vi "Add Units Panel 2.vi"(0 "System#":u8, 7 "Rack Number":i8=1 min=1 max=16, 8 "AutoAge.ini  File Path":path=path "\\\\Beco\\autoage/config/autoage.ini") -> ()   [LabVIEW 2021]
uses:
  Main Controls System v8.0/AutoAge Globals.vi
panel:
  out "Functional  Data":string
  out "title":string
  in  "Cancel":bool
  in  "Test":bool
  in  "Update":bool
  in  "Row33 to 40":bool
  in  "Row25 to 32":bool
  in  "Row17 to 24":bool
  in  "Row9 to 16":bool
  in  "Row1 to 8":bool
  in  "Select All":bool
  in  "40":bool
  in  "39":bool
  in  "38":bool
  in  "37":bool
  in  "36":bool
  in  "35":bool
  in  "34":bool
  in  "33":bool
  in  "32":bool
  in  "31":bool
  in  "30":bool
  in  "29":bool
  in  "28":bool
  in  "27":bool
  in  "26":bool
  in  "25":bool
  in  "24":bool
  in  "23":bool
  in  "22":bool
  in  "21":bool
  in  "20":bool
  in  "19":bool
  in  "18":bool
  in  "17":bool
  in  "16":bool
  in  "15":bool
  in  "14":bool
  in  "13":bool
  in  "12":bool
  in  "11":bool
  in  "10":bool
  in  "9":bool
  in  "8":bool
  in  "7":bool
  in  "6":bool
  in  "5":bool
  in  "4":bool
  in  "3":bool
  in  "2":bool
  in  "1":bool
  out "Rack":i8=1 min=1 max=16
  in  "Done":bool
  # "Click to turn on the inactive positions.  A red square   in a position indicates that a position is going to run."
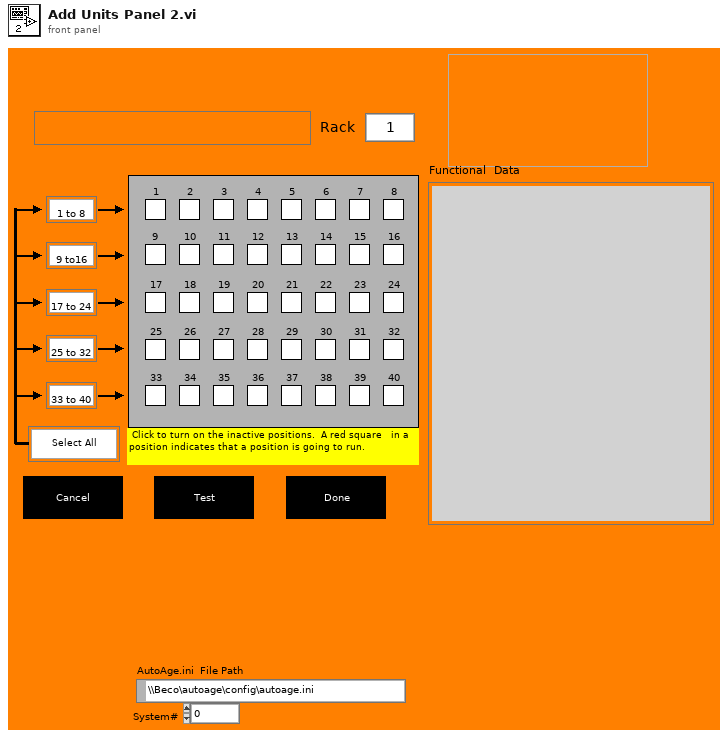
[diagram p1: front panel]
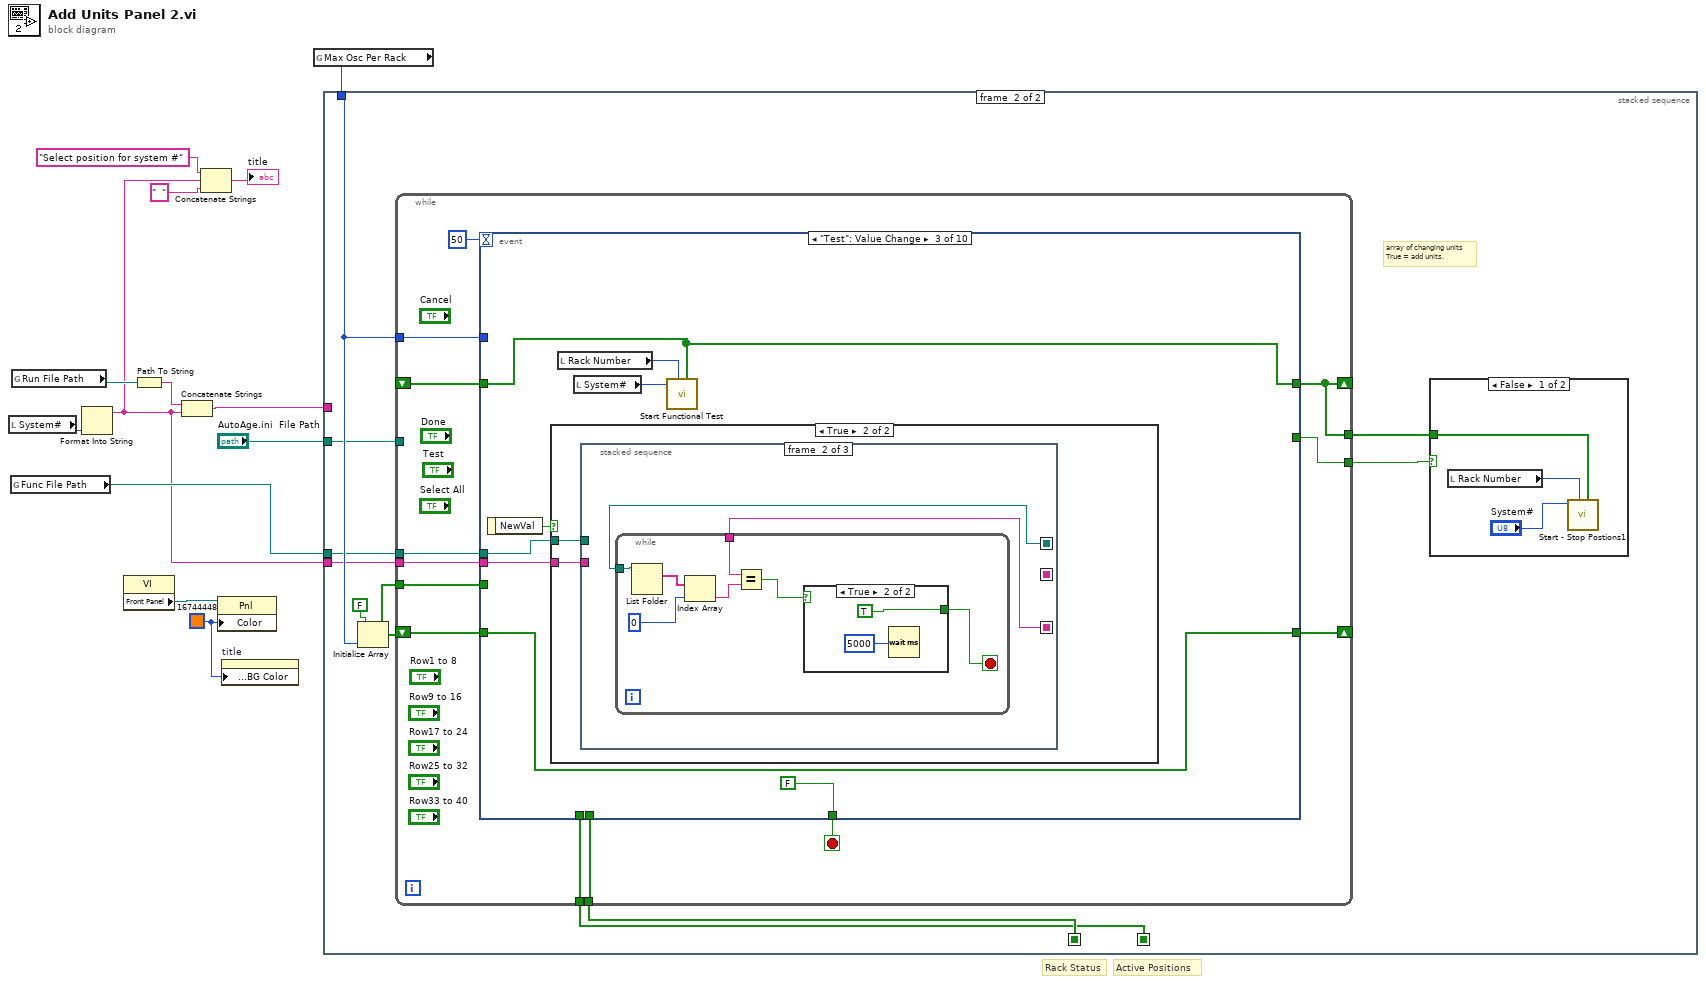
[diagram p0: block diagram]
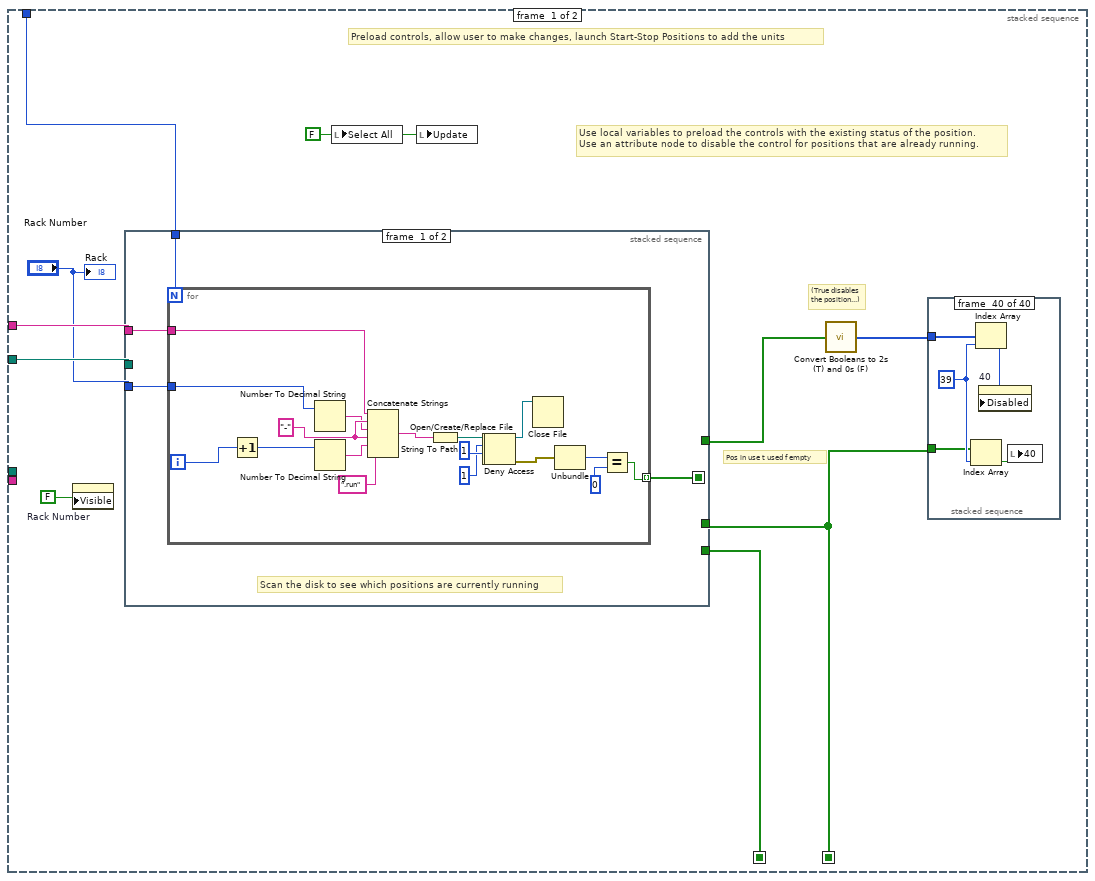
[diagram p2: hidden frame]
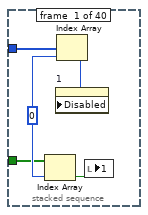
[diagram p3: hidden frame]
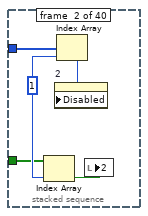
[diagram p4: hidden frame]
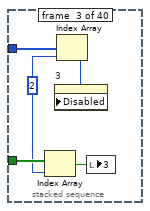
[diagram p5: hidden frame]
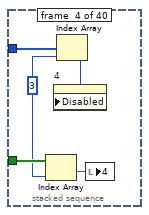
[diagram p6: hidden frame]
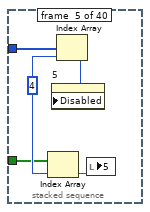
[diagram p7: hidden frame]
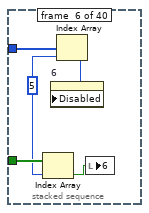
[diagram p8: hidden frame]
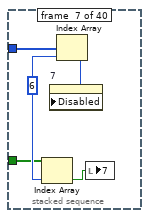
[diagram p9: hidden frame]
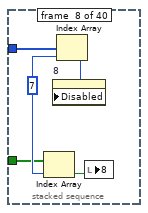
[diagram p10: hidden frame]
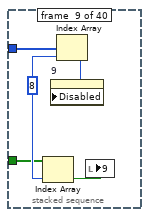
[diagram p11: hidden frame]
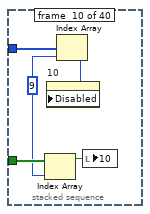
[diagram p12: hidden frame]
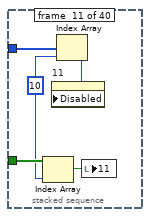
[diagram p13: hidden frame]
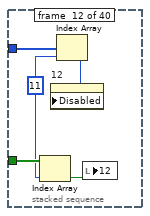
[diagram p14: hidden frame]
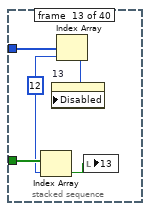
[diagram p15: hidden frame]
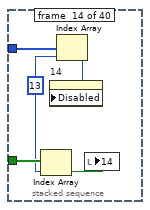
[diagram p16: hidden frame]
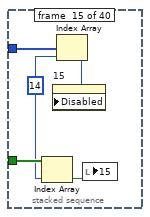
[diagram p17: hidden frame]
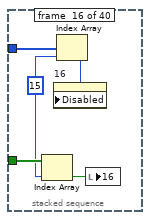
[diagram p18: hidden frame]
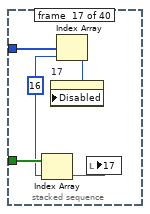
[diagram p19: hidden frame]
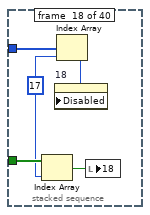
[diagram p20: hidden frame]
diagram:
  w1 = u32 16744448
  # "Active Positions"
  # "Rack Status"
  n1 = local read "System#"() -> (w11:u8)
  n2 = global read "AutoAge Globals.vi" "Func File Path"() -> (w7:path)
  n3 = global read "AutoAge Globals.vi" "Run File Path"() -> (w12:path)
  n4 = Format Into String(w11) -> (resulting string=w4:string)  [unwired: 3 in, 1 out]
  n5 = property class="VI"() -> ("Front Panel"=w6:refnum<vi>)  [unwired: 2 in, 2 out]
  n6 = Path To String(path=w12) -> (string=w8:string)
  n7 = Concatenate Strings(w8, w4) -> (w10:string)
  n8 = Concatenate Strings("Select position for system #", w4, "  ") -> (→"title":string)
  n9 = property class="Pnl"(reference=w6, "Color"=w1) -> ()  [unwired: 1 in, 2 out]
  n10 = property on="title" class="Str"("Text.Text Colors:BG Color"=w1) -> ()  [unwired: 2 in, 2 out]
  n11 = global read "AutoAge Globals.vi" "Max Osc Per Rack"() -> (w9:u16)
  n12 = stacked-sequence {
    seq-local: [w19 _] -> [_ w278]
    seq-local: [w14 _] -> [_ w279]
    tunnel: "AutoAge.ini  File Path" -> [w22 w273]
    tunnel: w10 -> [w21 _]
    tunnel: w9 -> [w17 w282]
    tunnel: w7 -> [_ w277]
    tunnel: w4 -> [_ w276]
    frame #0 {
      w16 = FALSE ("Select All")
      # "Pos in use t used f empty"
      # "(True disables\nthe position...)"
      # "Preload controls, allow user to make changes, launch Start-Stop Positions to add the units"
      # "Use local variables to preload the controls with the existing status of the position.\nUse an attribute node to disable the control for positions that are already running."
      n13 = property on="Rack Number" class="DigNum (strict)"("Visible"=FALSE) -> ()  [unwired: 2 in, 2 out]
      n14 = stacked-sequence {
        seq-local: [w227 _] -> [_ w253]
        tunnel: "Rack Number" -> [w226 w261]
        tunnel: [_ w252] -> w15
        tunnel: [_ w253] -> w19
        tunnel: w22 -> [_ w250]
        tunnel: w21 -> [w225 _]
        tunnel: w17 -> [w224 w249]
        tunnel: [_ w247] -> w14
        frame #0 {
          # "Scan the disk to see which positions are currently running"
          n15 = for {
            N: w224 -> [_]
            tunnel: [w231] -> w227 mode=indexing
            tunnel: w226 -> [w233]
            tunnel: w225 -> [w232]
            i -> [w230]
            w246 = "-"
            n16 = Increment(x=w230) -> (x+1=w244:i32)
            n17 = Number To Decimal String(number=w233) -> (decimal integer string=w241:string)  [unwired: 1 in]
            n18 = Number To Decimal String(number=w244) -> (decimal integer string=w242:string)  [unwired: 1 in]
            n19 = Concatenate Strings(w232, w246, w241, w246, w242, ".run") -> (w243:string)
            n20 = String To Path(string=w243) -> (path=w234:path)
            n21 = Open/Create/Replace File(file path (use dialog)=w234, access (0:read/write)=1) -> (refnum out=w228:refnum<file>, error out=w229:errorcluster)  [unwired: 4 in, 1 out]
            n22 = Deny Access(4:w229, 6:1, 7:w228) -> (0:w237:errorcluster, 3:w240:refnum<file>)
            n23 = Close File(refnum=w240) -> ()  [unwired: 1 in, 2 out]
            n24 = Unbundle(w237) -> ("code"=w239:i32)  [unwired: 2 out]
            n25 = Equal?(x=w239, y=0) -> (x = y?=w231:bool)
          }
        }
        frame #1 {
          # "default all pos false"
          # "Resolve card disabled"
          # "resolve rack enabled\nall pos false if disabled"
          # "Check configuration file to see which racks are disabled and how many cards are in each switcher"
          n26 = Decrement(x=w261) -> (x-1=w251:i8)
          n27 = call "Load Rack Config"("AutoAge.ini  File Path"=w250) -> ("Rack Status"=w262:string[], "# of Cards"=w266:i32[])  [unwired: 1 out]
          n28 = Index Array(array=w262, index=w251) -> (element=w260:string)
          n29 = Index Array(array=w266, index=w251) -> (element=w267:i32)
          n30 = Initialize Array(FALSE, w249) -> (w256:bool[])
          n31 = To Lower Case(string=w260) -> (all lower case string=w265:string)
          n32 = Multiply(x=w267, y=8) -> (x*y=w257:i32)
          n33 = for {
            N: w249 -> [_]
            tunnel: w257 -> [w272]
            shift-right: [w269] -> w254
            shift-left: w256 -> [w270]
            i -> [w268]
            n34 = Greater?(x=w272, y=w268) -> (0:w271:bool)
            n35 = Replace Array Subset(array=w270, new element=w271, index=w268) -> (w269:bool[])
          }
          n36 = Equal?(x=w265, y="enabled") -> (x = y?=w259:bool)
          n37 = Initialize Array(w259, w249) -> (w255:bool[])
          n38 = And(x=w255, y=w254) -> (x .and. y?=w247:bool[])
          n39 = Not(x=w247) -> (.not. x?=w248:bool[])
          n40 = Or(x=w248, y=w253) -> (x .or. y?=w252:bool[])
        }
      }
      n41 = local write "Select All"(w16) -> ()
      n42 = local write "Update"(w16) -> ()
      n43 = call "Convert Booleans to 2s (T) and 0s (F)"("Boolean Array"=w15) -> ("2s and 0s"=w18:u8[])
      n44 = stacked-sequence {
        tunnel: w18 -> [w28 w33 w38 w43 w48 w53 w58 w63 w68 w73 w78 w83 w88 w93 w98 w103 w108 w113 w118 w123 w128 w133 w138 w143 w148 w153 w158 w163 w168 w173 w178 w183 w188 w193 w198 w203 w208 w213 w218 w223]
        tunnel: w19 -> [w25 w30 w37 w42 w46 w52 w56 w61 w66 w72 w77 w82 w87 w92 w97 w102 w107 w112 w117 w122 w127 w132 w137 w142 w147 w152 w157 w162 w167 w172 w177 w182 w187 w192 w197 w202 w207 w212 w217 w220]
        frame #0 {
          w26 = 0
          n45 = Index Array(array=w25, index=w26) -> (element=w27:bool)
          n46 = Index Array(array=w28, index=w26) -> (element=w24:u8)
          n47 = property on="1" class="Bool (strict)"("Disabled"=w24) -> ()  [unwired: 2 in, 2 out]
          n48 = local write "1"(w27) -> ()
        }
        frame #1 {
          w32 = 1
          n49 = Index Array(array=w30, index=w32) -> (element=w31:bool)
          n50 = Index Array(array=w33, index=w32) -> (element=w29:u8)
          n51 = property on="2" class="Bool (strict)"("Disabled"=w29) -> ()  [unwired: 2 in, 2 out]
          n52 = local write "2"(w31) -> ()
        }
        frame #2 {
          w36 = 2
          n53 = Index Array(array=w37, index=w36) -> (element=w35:bool)
          n54 = Index Array(array=w38, index=w36) -> (element=w34:u8)
          n55 = property on="3" class="Bool (strict)"("Disabled"=w34) -> ()  [unwired: 2 in, 2 out]
          n56 = local write "3"(w35) -> ()
        }
        frame #3 {
          w41 = 3
          n57 = Index Array(array=w42, index=w41) -> (element=w40:bool)
          n58 = Index Array(array=w43, index=w41) -> (element=w39:u8)
          n59 = property on="4" class="Bool (strict)"("Disabled"=w39) -> ()  [unwired: 2 in, 2 out]
          n60 = local write "4"(w40) -> ()
        }
        frame #4 {
          w47 = 4
          n61 = Index Array(array=w46, index=w47) -> (element=w45:bool)
          n62 = Index Array(array=w48, index=w47) -> (element=w44:u8)
          n63 = property on="5" class="Bool (strict)"("Disabled"=w44) -> ()  [unwired: 2 in, 2 out]
          n64 = local write "5"(w45) -> ()
        }
        frame #5 {
          w51 = 5
          n65 = Index Array(array=w52, index=w51) -> (element=w50:bool)
          n66 = Index Array(array=w53, index=w51) -> (element=w49:u8)
          n67 = property on="6" class="Bool (strict)"("Disabled"=w49) -> ()  [unwired: 2 in, 2 out]
          n68 = local write "6"(w50) -> ()
        }
        frame #6 {
          w57 = 6
          n69 = Index Array(array=w56, index=w57) -> (element=w55:bool)
          n70 = Index Array(array=w58, index=w57) -> (element=w54:u8)
          n71 = property on="7" class="Bool (strict)"("Disabled"=w54) -> ()  [unwired: 2 in, 2 out]
          n72 = local write "7"(w55) -> ()
        }
        frame #7 {
          w62 = 7
          n73 = Index Array(array=w61, index=w62) -> (element=w60:bool)
          n74 = Index Array(array=w63, index=w62) -> (element=w59:u8)
          n75 = property on="8" class="Bool (strict)"("Disabled"=w59) -> ()  [unwired: 2 in, 2 out]
          n76 = local write "8"(w60) -> ()
        }
        frame #8 {
          w67 = 8
          n77 = Index Array(array=w66, index=w67) -> (element=w65:bool)
          n78 = Index Array(array=w68, index=w67) -> (element=w64:u8)
          n79 = property on="9" class="Bool (strict)"("Disabled"=w64) -> ()  [unwired: 2 in, 2 out]
          n80 = local write "9"(w65) -> ()
        }
        frame #9 {
          w70 = 9
          n81 = Index Array(array=w72, index=w70) -> (element=w71:bool)
          n82 = Index Array(array=w73, index=w70) -> (element=w69:u8)
          n83 = property on="10" class="Bool (strict)"("Disabled"=w69) -> ()  [unwired: 2 in, 2 out]
          n84 = local write "10"(w71) -> ()
        }
        frame #10 {
          w75 = 10
          n85 = Index Array(array=w77, index=w75) -> (element=w76:bool)
          n86 = Index Array(array=w78, index=w75) -> (element=w74:u8)
          n87 = property on="11" class="Bool (strict)"("Disabled"=w74) -> ()  [unwired: 2 in, 2 out]
          n88 = local write "11"(w76) -> ()
        }
        frame #11 {
          w80 = 11
          n89 = Index Array(array=w82, index=w80) -> (element=w81:bool)
          n90 = Index Array(array=w83, index=w80) -> (element=w79:u8)
          n91 = property on="12" class="Bool (strict)"("Disabled"=w79) -> ()  [unwired: 2 in, 2 out]
          n92 = local write "12"(w81) -> ()
        }
        frame #12 {
          w85 = 12
          n93 = Index Array(array=w87, index=w85) -> (element=w86:bool)
          n94 = Index Array(array=w88, index=w85) -> (element=w84:u8)
          n95 = property on="13" class="Bool (strict)"("Disabled"=w84) -> ()  [unwired: 2 in, 2 out]
          n96 = local write "13"(w86) -> ()
        }
        frame #13 {
          w91 = 13
          n97 = Index Array(array=w92, index=w91) -> (element=w90:bool)
          n98 = Index Array(array=w93, index=w91) -> (element=w89:u8)
          n99 = property on="14" class="Bool (strict)"("Disabled"=w89) -> ()  [unwired: 2 in, 2 out]
          n100 = local write "14"(w90) -> ()
        }
        frame #14 {
          w96 = 14
          n101 = Index Array(array=w97, index=w96) -> (element=w95:bool)
          n102 = Index Array(array=w98, index=w96) -> (element=w94:u8)
          n103 = property on="15" class="Bool (strict)"("Disabled"=w94) -> ()  [unwired: 2 in, 2 out]
          n104 = local write "15"(w95) -> ()
        }
        frame #15 {
          w101 = 15
          n105 = Index Array(array=w102, index=w101) -> (element=w100:bool)
          n106 = Index Array(array=w103, index=w101) -> (element=w99:u8)
          n107 = property on="16" class="Bool (strict)"("Disabled"=w99) -> ()  [unwired: 2 in, 2 out]
          n108 = local write "16"(w100) -> ()
        }
        frame #16 {
          w106 = 16
          n109 = Index Array(array=w107, index=w106) -> (element=w105:bool)
          n110 = Index Array(array=w108, index=w106) -> (element=w104:u8)
          n111 = property on="17" class="Bool (strict)"("Disabled"=w104) -> ()  [unwired: 2 in, 2 out]
          n112 = local write "17"(w105) -> ()
        }
        frame #17 {
          w111 = 17
          n113 = Index Array(array=w112, index=w111) -> (element=w110:bool)
          n114 = Index Array(array=w113, index=w111) -> (element=w109:u8)
          n115 = property on="18" class="Bool (strict)"("Disabled"=w109) -> ()  [unwired: 2 in, 2 out]
          n116 = local write "18"(w110) -> ()
        }
        frame #18 {
          w116 = 18
          n117 = Index Array(array=w117, index=w116) -> (element=w115:bool)
          n118 = Index Array(array=w118, index=w116) -> (element=w114:u8)
          n119 = property on="19" class="Bool (strict)"("Disabled"=w114) -> ()  [unwired: 2 in, 2 out]
          n120 = local write "19"(w115) -> ()
        }
        frame #19 {
          w121 = 19
          n121 = Index Array(array=w122, index=w121) -> (element=w120:bool)
          n122 = Index Array(array=w123, index=w121) -> (element=w119:u8)
          n123 = property on="20" class="Bool (strict)"("Disabled"=w119) -> ()  [unwired: 2 in, 2 out]
          n124 = local write "20"(w120) -> ()
        }
        frame #20 {
          w125 = 20
          n125 = Index Array(array=w127, index=w125) -> (element=w126:bool)
          n126 = Index Array(array=w128, index=w125) -> (element=w124:u8)
          n127 = property on="21" class="Bool (strict)"("Disabled"=w124) -> ()  [unwired: 2 in, 2 out]
          n128 = local write "21"(w126) -> ()
        }
        frame #21 {
          w131 = 21
          n129 = Index Array(array=w132, index=w131) -> (element=w130:bool)
          n130 = Index Array(array=w133, index=w131) -> (element=w129:u8)
          n131 = property on="22" class="Bool (strict)"("Disabled"=w129) -> ()  [unwired: 2 in, 2 out]
          n132 = local write "22"(w130) -> ()
        }
        frame #22 {
          w136 = 22
          n133 = Index Array(array=w137, index=w136) -> (element=w135:bool)
          n134 = Index Array(array=w138, index=w136) -> (element=w134:u8)
          n135 = property on="23" class="Bool (strict)"("Disabled"=w134) -> ()  [unwired: 2 in, 2 out]
          n136 = local write "23"(w135) -> ()
        }
        frame #23 {
          w141 = 23
          n137 = Index Array(array=w142, index=w141) -> (element=w140:bool)
          n138 = Index Array(array=w143, index=w141) -> (element=w139:u8)
          n139 = property on="24" class="Bool (strict)"("Disabled"=w139) -> ()  [unwired: 2 in, 2 out]
          n140 = local write "24"(w140) -> ()
        }
        frame #24 {
          w146 = 24
          n141 = Index Array(array=w147, index=w146) -> (element=w145:bool)
          n142 = Index Array(array=w148, index=w146) -> (element=w144:u8)
          n143 = property on="25" class="Bool (strict)"("Disabled"=w144) -> ()  [unwired: 2 in, 2 out]
          n144 = local write "25"(w145) -> ()
        }
        frame #25 {
          w151 = 25
          n145 = Index Array(array=w152, index=w151) -> (element=w150:bool)
          n146 = Index Array(array=w153, index=w151) -> (element=w149:u8)
          n147 = property on="26" class="Bool (strict)"("Disabled"=w149) -> ()  [unwired: 2 in, 2 out]
          n148 = local write "26"(w150) -> ()
        }
        frame #26 {
          w156 = 26
          n149 = Index Array(array=w157, index=w156) -> (element=w155:bool)
          n150 = Index Array(array=w158, index=w156) -> (element=w154:u8)
          n151 = property on="27" class="Bool (strict)"("Disabled"=w154) -> ()  [unwired: 2 in, 2 out]
          n152 = local write "27"(w155) -> ()
        }
        frame #27 {
          w161 = 27
          n153 = Index Array(array=w162, index=w161) -> (element=w160:bool)
          n154 = Index Array(array=w163, index=w161) -> (element=w159:u8)
          n155 = property on="28" class="Bool (strict)"("Disabled"=w159) -> ()  [unwired: 2 in, 2 out]
          n156 = local write "28"(w160) -> ()
        }
        frame #28 {
          w166 = 28
          n157 = Index Array(array=w167, index=w166) -> (element=w165:bool)
          n158 = Index Array(array=w168, index=w166) -> (element=w164:u8)
          n159 = property on="29" class="Bool (strict)"("Disabled"=w164) -> ()  [unwired: 2 in, 2 out]
          n160 = local write "29"(w165) -> ()
        }
        frame #29 {
          w171 = 29
          n161 = Index Array(array=w172, index=w171) -> (element=w170:bool)
          n162 = Index Array(array=w173, index=w171) -> (element=w169:u8)
          n163 = property on="30" class="Bool (strict)"("Disabled"=w169) -> ()  [unwired: 2 in, 2 out]
          n164 = local write "30"(w170) -> ()
        }
        frame #30 {
          w176 = 30
          n165 = Index Array(array=w177, index=w176) -> (element=w175:bool)
          n166 = Index Array(array=w178, index=w176) -> (element=w174:u8)
          n167 = property on="31" class="Bool (strict)"("Disabled"=w174) -> ()  [unwired: 2 in, 2 out]
          n168 = local write "31"(w175) -> ()
        }
        frame #31 {
          w181 = 31
          n169 = Index Array(array=w182, index=w181) -> (element=w180:bool)
          n170 = Index Array(array=w183, index=w181) -> (element=w179:u8)
          n171 = property on="32" class="Bool (strict)"("Disabled"=w179) -> ()  [unwired: 2 in, 2 out]
          n172 = local write "32"(w180) -> ()
        }
        frame #32 {
          w186 = 32
          n173 = Index Array(array=w187, index=w186) -> (element=w185:bool)
          n174 = Index Array(array=w188, index=w186) -> (element=w184:u8)
          n175 = property on="33" class="Bool (strict)"("Disabled"=w184) -> ()  [unwired: 2 in, 2 out]
          n176 = local write "33"(w185) -> ()
        }
        frame #33 {
          w191 = 33
          n177 = Index Array(array=w192, index=w191) -> (element=w190:bool)
          n178 = Index Array(array=w193, index=w191) -> (element=w189:u8)
          n179 = property on="34" class="Bool (strict)"("Disabled"=w189) -> ()  [unwired: 2 in, 2 out]
          n180 = local write "34"(w190) -> ()
        }
        frame #34 {
          w196 = 34
          n181 = Index Array(array=w197, index=w196) -> (element=w195:bool)
          n182 = Index Array(array=w198, index=w196) -> (element=w194:u8)
          n183 = property on="35" class="Bool (strict)"("Disabled"=w194) -> ()  [unwired: 2 in, 2 out]
          n184 = local write "35"(w195) -> ()
        }
        frame #35 {
          w201 = 35
          n185 = Index Array(array=w202, index=w201) -> (element=w200:bool)
          n186 = Index Array(array=w203, index=w201) -> (element=w199:u8)
          n187 = property on="36" class="Bool (strict)"("Disabled"=w199) -> ()  [unwired: 2 in, 2 out]
          n188 = local write "36"(w200) -> ()
        }
        frame #36 {
          w206 = 36
          n189 = Index Array(array=w207, index=w206) -> (element=w205:bool)
          n190 = Index Array(array=w208, index=w206) -> (element=w204:u8)
          n191 = property on="37" class="Bool (strict)"("Disabled"=w204) -> ()  [unwired: 2 in, 2 out]
          n192 = local write "37"(w205) -> ()
        }
        frame #37 {
          w211 = 37
          n193 = Index Array(array=w212, index=w211) -> (element=w210:bool)
          n194 = Index Array(array=w213, index=w211) -> (element=w209:u8)
          n195 = property on="38" class="Bool (strict)"("Disabled"=w209) -> ()  [unwired: 2 in, 2 out]
          n196 = local write "38"(w210) -> ()
        }
        frame #38 {
          w216 = 38
          n197 = Index Array(array=w217, index=w216) -> (element=w215:bool)
          n198 = Index Array(array=w218, index=w216) -> (element=w214:u8)
          n199 = property on="39" class="Bool (strict)"("Disabled"=w214) -> ()  [unwired: 2 in, 2 out]
          n200 = local write "39"(w215) -> ()
        }
        frame #39 {
          w221 = 39
          n201 = Index Array(array=w220, index=w221) -> (element=w222:bool)
          n202 = Index Array(array=w223, index=w221) -> (element=w219:u8)
          n203 = property on="40" class="Bool (strict)"("Disabled"=w219) -> ()  [unwired: 2 in, 2 out]
          n204 = local write "40"(w222) -> ()
        }
      }
      "Rack" <- "Rack Number"
    }
    frame #1 {
      # "array of changing units\nTrue = add units."
      n205 = Initialize Array(FALSE, w282) -> (w280:bool[])
      n206 = while {
        tunnel: [w289] -> w274
        tunnel: w282 -> [w296]
        tunnel: w279 -> [w297]
        shift-right: [w289] -> _
        shift-left: _ -> [w294]
        shift-right: [w291] -> _
        shift-left: w280 -> [w293]
        tunnel: w280 -> [w292]
        tunnel: w278 -> [w290]
        tunnel: w277 -> [w288]
        tunnel: w276 -> [w287]
        tunnel: [w286] -> w275
        tunnel: w273 -> [_]
        stop <- w295 stop-if-true
        n207 = event shown="[2] \"Test\": Value Change" {
          selector: _ -> [_ _ _ _ _ _ _ _ _ _]
          dyn-events: _ -> [_ _ _ _ _ _ _ _ _ _]
          timeout: 50 -> [_ _ _ _ _ _ _ _ _ _]
          tunnel: [w300 w406 w414 _ _ _ _ _ w509 _] -> w289
          tunnel: w297 -> [w303 _ _ w451 w462 w473 w484 w495 _ _]
          tunnel: w296 -> [w301 w400 _ _ _ _ _ _ _ _]
          tunnel: [FALSE FALSE FALSE FALSE ("NewVal") FALSE ("NewVal") FALSE ("NewVal") FALSE FALSE w506 TRUE] -> w295
          tunnel: w294 -> [_ w406 w414 _ _ _ _ _ w509 _]
          tunnel: w293 -> [w302 w405 w413 w456 w466 w477 w489 w500 w508 _]
          tunnel: w292 -> [_ w404 _ _ _ _ _ _ _ _]
          tunnel: [w300 w401 w413 w452 w465 w476 w488 w499 w508 _] -> w291
          tunnel: w290 -> [w299 w399 _ _ _ _ _ _ _ _]
          tunnel: w288 -> [_ _ w415 _ _ _ _ _ _ _]
          tunnel: w287 -> [_ _ w419 _ _ _ _ _ _ _]
          tunnel: [_ _ _ _ _ _ _ _ FALSE w511] -> w286
          event Timeout {
            n208 = event-data() -> ()  [unwired: 1 in, 1 out]
            n209 = case shown="True" "Update" {
              tunnel: [w346 w349] -> w300
              tunnel: w303 -> [_ w352]
              tunnel: w302 -> [_ w351]
              tunnel: w301 -> [_ w350]
              tunnel: w299 -> [_ w347]
              frame False {
                # "The actual controls"
                n210 = Build Array("1", "2", "3", "4", "5", "6", "7", "8", "9", "10", "11", "12", "13", "14", "15", "16", "17", "18", "19", "20", "21", "22", "23", "24", "25", "26", "27", "28", "29", "30", "31", "32", "33", "34", "35", "36", "37", "38", "39", "40") -> (w346:bool[])
              }
              frame True {
                # "Loop changes list"
                # "true = enabled"
                # "true if run running"
                # "Update the Control Status"
                n211 = for {
                  N: w350 -> [_]
                  tunnel: w352 -> [w357] mode=indexing
                  tunnel: w351 -> [w356] mode=indexing
                  tunnel: [w354] -> w349 mode=indexing
                  tunnel: w347 -> [w353] mode=indexing
                  i -> [w358]
                  n212 = And(x=w357, y=w356) -> (x .and. y?=w355:bool)
                  n213 = Or(x=w353, y=w355) -> (x .or. y?=w354:bool)
                  n214 = case shown="39" w358 {
                    tunnel: w354 -> [w359 w360 w361 w362 w363 w364 w365 w366 w367 w368 w369 w370 w371 w372 w373 w374 w375 w376 w377 w378 w379 w380 w381 w382 w383 w384 w385 w386 w387 w388 w389 w390 w391 w392 w393 w394 w395 w396 w397 w398]
                    frame 0, Default {
                      n215 = local write "1"(w359) -> ()
                    }
                    frame 1 {
                      n216 = local write "2"(w360) -> ()
                    }
                    frame 2 {
                      n217 = local write "3"(w361) -> ()
                    }
                    frame 3 {
                      n218 = local write "4"(w362) -> ()
                    }
                    frame 4 {
                      n219 = local write "5"(w363) -> ()
                    }
                    frame 5 {
                      n220 = local write "6"(w364) -> ()
                    }
                    frame 6 {
                      n221 = local write "7"(w365) -> ()
                    }
                    frame 7 {
                      n222 = local write "8"(w366) -> ()
                    }
                    frame 8 {
                      n223 = local write "9"(w367) -> ()
                    }
                    frame 9 {
                      n224 = local write "10"(w368) -> ()
                    }
                    frame 10 {
                      n225 = local write "11"(w369) -> ()
                    }
                    frame 11 {
                      n226 = local write "12"(w370) -> ()
                    }
                    frame 12 {
                      n227 = local write "13"(w371) -> ()
                    }
                    frame 13 {
                      n228 = local write "14"(w372) -> ()
                    }
                    frame 14 {
                      n229 = local write "15"(w373) -> ()
                    }
                    frame 15 {
                      n230 = local write "16"(w374) -> ()
                    }
                    frame 16 {
                      n231 = local write "17"(w375) -> ()
                    }
                    frame 17 {
                      n232 = local write "18"(w376) -> ()
                    }
                    frame 18 {
                      n233 = local write "19"(w377) -> ()
                    }
                    frame 19 {
                      n234 = local write "20"(w378) -> ()
                    }
                    frame 20 {
                      n235 = local write "21"(w379) -> ()
                    }
                    frame 21 {
                      n236 = local write "22"(w380) -> ()
                    }
                    frame 22 {
                      n237 = local write "23"(w381) -> ()
                    }
                    frame 23 {
                      n238 = local write "24"(w382) -> ()
                    }
                    frame 24 {
                      n239 = local write "25"(w383) -> ()
                    }
                    frame 25 {
                      n240 = local write "26"(w384) -> ()
                    }
                    frame 26 {
                      n241 = local write "27"(w385) -> ()
                    }
                    frame 27 {
                      n242 = local write "28"(w386) -> ()
                    }
                    frame 28 {
                      n243 = local write "29"(w387) -> ()
                    }
                    frame 29 {
                      n244 = local write "30"(w388) -> ()
                    }
                    frame 30 {
                      n245 = local write "31"(w389) -> ()
                    }
                    frame 31 {
                      n246 = local write "32"(w390) -> ()
                    }
                    frame 32 {
                      n247 = local write "33"(w391) -> ()
                    }
                    frame 33 {
                      n248 = local write "34"(w392) -> ()
                    }
                    frame 34 {
                      n249 = local write "35"(w393) -> ()
                    }
                    frame 35 {
                      n250 = local write "36"(w394) -> ()
                    }
                    frame 36 {
                      n251 = local write "37"(w395) -> ()
                    }
                    frame 37 {
                      n252 = local write "38"(w396) -> ()
                    }
                    frame 38 {
                      n253 = local write "39"(w397) -> ()
                    }
                    frame 39 {
                      n254 = local write "40"(w398) -> ()
                    }
                  }
                }
                n255 = local write "Update"(FALSE ("Update")) -> ()
              }
            }
          }
          event "Select All": Value Change {
            n256 = event-data() -> ("NewVal"=w402:bool)  [unwired: 1 in]
            n257 = case shown="False" w402 {
              tunnel: w405 -> [w408 w409]
              tunnel: w404 -> [_ _]
              tunnel: [w408 w412] -> w401
              tunnel: w399 -> [_ w410]
              tunnel: w400 -> [_ w411]
              frame False {
              }
              frame True {
                n258 = call "Select All Status.vi"("Max Positions per Rack"=w411, "Active Positions"=w409, "Rack Status In"=w410) -> ("Rack Status Out"=w412:bool[])
              }
            }
            n259 = local write "Update"(TRUE ("Update")) -> ()
          }
          event "Test": Value Change {
            n260 = event-data() -> ("NewVal"=w420:bool)  [unwired: 1 in]
            n261 = case shown="True" w420 {
              tunnel: w419 -> [_ w422]
              tunnel: w415 -> [_ w421]
              frame False {
              }
              frame True {
                n262 = stacked-sequence {
                  seq-local: [w425 _ _] -> [_ w434 _]
                  seq-local: [w426 _ _] -> [_ _ w446]
                  seq-local: [w423 _ _] -> [_ w433 _]
                  tunnel: w422 -> [w427 _ _]
                  tunnel: w421 -> [w424 _ _]
                  frame #0 {
                    n263 = Path To String(path=w424) -> (string=w428:string)
                    n264 = Concatenate Strings(w428, w427) -> (w430:string)
                    n265 = Concatenate Strings("func", w427, ".rslt") -> (w423:string)
                    n266 = String To Path(string=w430) -> (path=w425:path)
                    n267 = Concatenate Strings(w430, "\\", w423) -> (w426:string)
                  }
                  frame #1 {
                    n268 = while {
                      tunnel: w434 -> [w441]
                      tunnel: w433 -> [w435]
                      stop <- w436 stop-if-true
                      n269 = List Folder(path=w441) -> (filenames=w439:string[])  [unwired: 3 in, 3 out]
                      n270 = Index Array(array=w439, index=0) -> (element=w438:string)
                      n271 = Equal?(x=w435, y=w438) -> (x = y?=w437:bool)
                      n272 = case shown="True" w437 {
                        tunnel: [FALSE TRUE] -> w436
                        frame False {
                          n273 = Wait (ms)(milliseconds to wait=100) -> ()  [unwired: 1 out]
                        }
                        frame True {
                          n274 = Wait (ms)(milliseconds to wait=5000) -> ()  [unwired: 1 out]
                        }
                      }
                    }
                  }
                  frame #2 {
                    n275 = String To Path(string=w446) -> (path=w448:path)
                    n276 = call <vilib>:"Read Lines From File.vi"("file path (dialog if empty)"=w448, "number of lines (all:-1)"=-1) -> ("new file path (Not A Path if cancelled)"=w447:path, "line string"=→"Functional  Data":string)  [unwired: 4 in, 2 out]
                    n277 = Delete(path (use dialog)=w447) -> ()  [unwired: 4 in, 3 out]
                  }
                }
              }
            }
            n278 = local read "Rack Number"() -> (w416:i8)
            n279 = local read "System#"() -> (w417:u8)
            n280 = call "Start Functional Test.vi"("New Status of Positions"=w414, "Rack Number"=w416, "System#"=w417) -> ()  [unwired: 9 in]
          }
          event "Row1 to 8": Value Change {
            n281 = event-data() -> ("NewVal"=w455:bool)  [unwired: 1 in]
            n282 = case shown="True" w455 {
              tunnel: w456 -> [w457 w461]
              tunnel: [w457 w460] -> w452
              tunnel: w451 -> [_ w458]
              frame False {
              }
              frame True {
                n283 = call "Check Current Row Status.vi"("Row"=1, "Active Positions"=w458, "Rack Status In"=w461) -> ("Rack Status Out"=w460:bool[])
              }
            }
            n284 = local write "Update"(TRUE ("Update")) -> ()
          }
          event "Row9 to 16": Value Change {
            n285 = event-data() -> ("NewVal"=w467:bool)  [unwired: 1 in]
            n286 = case shown="True" w467 {
              tunnel: w466 -> [w468 w472]
              tunnel: [w468 w471] -> w465
              tunnel: w462 -> [_ w469]
              frame False {
              }
              frame True {
                n287 = call "Check Current Row Status.vi"("Row"=2, "Active Positions"=w469, "Rack Status In"=w472) -> ("Rack Status Out"=w471:bool[])
              }
            }
            n288 = local write "Update"(TRUE ("Update")) -> ()
          }
          event "Row17 to 24": Value Change {
            n289 = event-data() -> ("NewVal"=w478:bool)  [unwired: 1 in]
            n290 = case shown="True" w478 {
              tunnel: w477 -> [w479 w483]
              tunnel: [w479 w482] -> w476
              tunnel: w473 -> [_ w480]
              frame False {
              }
              frame True {
                n291 = call "Check Current Row Status.vi"("Row"=3, "Active Positions"=w480, "Rack Status In"=w483) -> ("Rack Status Out"=w482:bool[])
              }
            }
            n292 = local write "Update"(TRUE ("Update")) -> ()
          }
          event "Row25 to 32": Value Change {
            n293 = event-data() -> ("NewVal"=w487:bool)  [unwired: 1 in]
            n294 = case shown="True" w487 {
              tunnel: w489 -> [w490 w494]
              tunnel: [w490 w493] -> w488
              tunnel: w484 -> [_ w491]
              frame False {
              }
              frame True {
                n295 = call "Check Current Row Status.vi"("Row"=4, "Active Positions"=w491, "Rack Status In"=w494) -> ("Rack Status Out"=w493:bool[])
              }
            }
            n296 = local write "Update"(TRUE ("Update")) -> ()
          }
          event "Row33 to 40": Value Change {
            n297 = event-data() -> ("NewVal"=w498:bool)  [unwired: 1 in]
            n298 = case shown="True" w498 {
              tunnel: w500 -> [w501 w505]
              tunnel: [w501 w504] -> w499
              tunnel: w495 -> [_ w502]
              frame False {
              }
              frame True {
                n299 = call "Check Current Row Status.vi"("Row"=5, "Active Positions"=w502, "Rack Status In"=w505) -> ("Rack Status Out"=w504:bool[])
              }
            }
            n300 = local write "Update"(TRUE ("Update")) -> ()
          }
          event "Done": Value Change {
            n301 = event-data() -> ("NewVal"=w506:bool)  [unwired: 1 in]
          }
          event "Cancel": Value Change {
            n302 = event-data() -> ("NewVal"=w511:bool)  [unwired: 1 in]
          }
        }
      }
      n303 = case shown="False" w275 {
        tunnel: w274 -> [w283 _]
        frame False {
          n304 = local read "Rack Number"() -> (w284:i8)
          n305 = call "Start - Stop Postions1.vi"("New Status of Positions"=w283, "Rack Number"=w284, "System#"="System#") -> ()  [unwired: 9 in]
        }
        frame True {
        }
      }
    }
  }
